vi "StartTransaction.vi"(8 "ErrorIn":errorcluster caption="Error In(no Error)", 11 "ReferenceIn":refnum<class "ErrorDefinitionSQLite.lvclass"> caption="Reference In") -> (0 "ErrorOut":errorcluster caption="Error Out", 1 "NIGUID":string, 3 "ReferenceOut":refnum<class "ErrorDefinitionSQLite.lvclass"> caption="Reference Out")   [LabVIEW 2021, in "ErrorDefinitionSQLite.lvclass"]
uses:
  ErrorDefinitionSQLite.lvclass
  <vilib>/drjdpowell/SQLite Library/Transaction Helpers/Transaction.lvlib
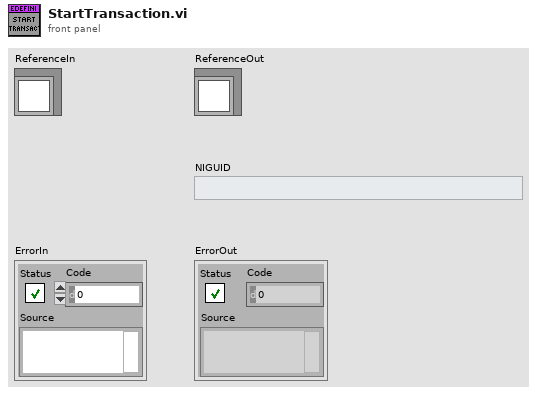
[diagram p1: front panel]
types:
  T1 = typedef "ErrorDefinitionSQLite.lvclass/ObjectAttributes.ctl" = cluster{"Path":path, "SQLiteRef":refnum<class "Connection.lvclass">, "EndOfRange":i32, "StartOfRange":i32}
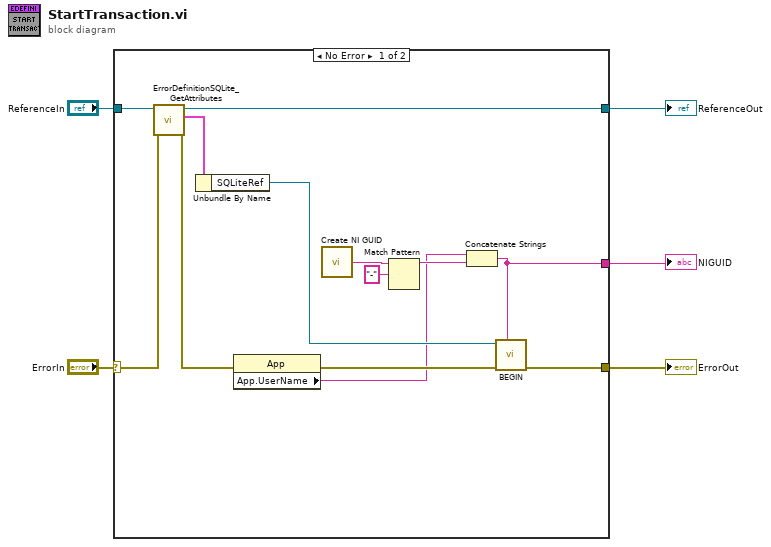
[diagram p0: block diagram]
diagram:
  n1 = case shown="No Error" "ErrorIn" {
    selector: "ErrorIn" -> [w18 w20]
    tunnel: [w17 w20] -> w4
    tunnel: [w13 w19] -> w2
    tunnel: "ReferenceIn" -> [w14 w19]
    tunnel: [w7 _] -> w1
    frame No Error {
      n2 = call "ErrorDefinitionSQLite_GetAttributes.vi"("ErrorIn"=w18, "ReferenceIn"=w14) -> ("ErrorOut"=w16:errorcluster, "Data"=w12:T1, "ReferenceOut"=w13:refnum<class "ErrorDefinitionSQLite.lvclass">)  [unwired: 6 in, 1 out]
      n3 = Unbundle By Name(w12) -> ("SQLiteRef"=w11:refnum<class "Connection.lvclass">)
      n4 = property class="App"(error in=w16) -> (error out=w15:errorcluster, "App.UserName"=w6:string)  [unwired: 1 in, 1 out]
      n5 = call <vilib>:"Create NI GUID.vi"() -> ("NI GUID"=w10:string)
      n6 = Match Pattern(string=w10, regular expression="-") -> (before substring=w9:string)  [unwired: 1 in, 3 out]
      n7 = Concatenate Strings(w6, w9) -> (w7:string)
      n8 = call <vilib>:"BEGIN.vi"("Savepoint name"=w7, "error in (no error)"=w15, "SQLite Connection in"=w11) -> ("error out"=w17:errorcluster)  [unwired: 7 in, 1 out]
    }
    frame Error {
    }
  }
  "ErrorOut" <- w4
  "ReferenceOut" <- w2
  "NIGUID" <- w1
